vi "Text time to numeric.vi"(1 "Time text input":string) -> (0 "Time numeric output":ext format="%.5f")   [LabVIEW 2015]
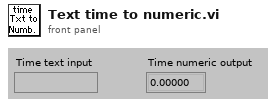
[diagram p1: front panel]
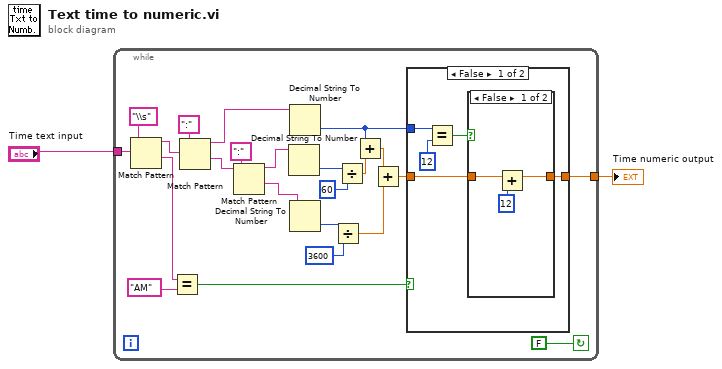
[diagram p0: block diagram]
diagram:
  n1 = while {
    tunnel: "Time text input" -> [w25]
    tunnel: [w6] -> w2
    stop <- FALSE continue-if-true
    n2 = Match Pattern(string=w25, regular expression="\\s") -> (before substring=w23:string, after substring=w9:string)  [unwired: 1 in, 2 out]
    n3 = Equal?(x=w9, y="AM") -> (x = y?=w7:bool)
    n4 = Match Pattern(string=w23, regular expression=":") -> (before substring=w21:string, after substring=w20:string)  [unwired: 1 in, 2 out]
    n5 = Match Pattern(string=w20, regular expression=":") -> (before substring=w18:string, after substring=w17:string)  [unwired: 1 in, 2 out]
    n6 = Decimal String To Number(string=w18) -> (number=w16:i32)  [unwired: 2 in, 1 out]
    n7 = Decimal String To Number(string=w21) -> (number=w4:i32)  [unwired: 2 in, 1 out]
    n8 = Decimal String To Number(string=w17) -> (number=w12:i32)  [unwired: 2 in, 1 out]
    n9 = Divide(x=w12, y=3600) -> (x/y=w10:dbl)
    n10 = Divide(x=w16, y=60) -> (x/y=w14:dbl)
    n11 = Add(x=w4, y=w14) -> (x+y=w13:dbl)
    n12 = Add(x=w13, y=w10) -> (x+y=w5:dbl)
    n13 = case shown="False" w7 {
      tunnel: w5 -> [w30 w35]
      tunnel: [w29 w35] -> w6
      tunnel: w4 -> [w28 _]
      frame False {
        n14 = Equal?(x=w28, y=12) -> (x = y?=w27:bool)
        n15 = case shown="False" w27 {
          tunnel: [w33 w34] -> w29
          tunnel: w30 -> [w31 w34]
          frame False {
            n16 = Add(x=w31, y=12) -> (x+y=w33:dbl)
          }
          frame True {
          }
        }
      }
      frame True {
      }
    }
  }
  "Time numeric output" <- w2
